vi "Excel_Insert_Control.vi"(0 "Worksheet":refnum<k7>, 1 "Excel.Shapes":refnum<k7>, 5 "Ctl Refnum":refnum<vi>, 7 "image depth":T1=3 items=["B&W", "4 bits", "8 bits", "24 bits"], 9 "image file type(.jpg)":enum16{".jpg", ".png"}(ring), 11 "error in (no error)":errorcluster, 12 "Position (Excel)":cluster{"row":i32, "column":i32}, 13 "name":string) -> (15 "error out":errorcluster)   [LabVIEW 2017, in "NI_ReportGenerationToolkit.lvlib"]
uses:
  <vilib>/addons/_office/NI_ReportGenerationToolkit.lvlib
  <vilib>/Utility/NIReport.llb/image depth.ctl
  <vilib>/Utility/NIReport.llb/NI_ReportGenerationCore.lvlib
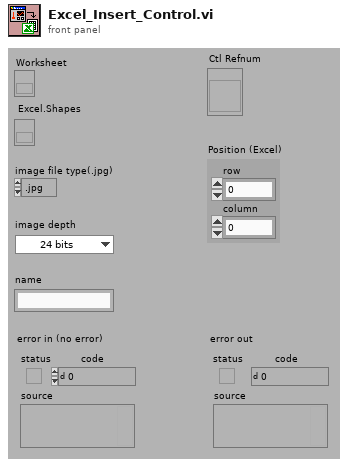
[diagram p1: front panel]
types:
  T1 = typedef "NI_ReportGenerationCore.lvlib/image depth.ctl" = u16
  T2 = typedef "imagedata.ctl" = cluster{"image type":i32, "image depth":i32, "image":u8[], "mask":u8[], "colors":u32[], "Rectangle":cluster{"left":i16, "top":i16, "right":i16, "bottom":i16}}
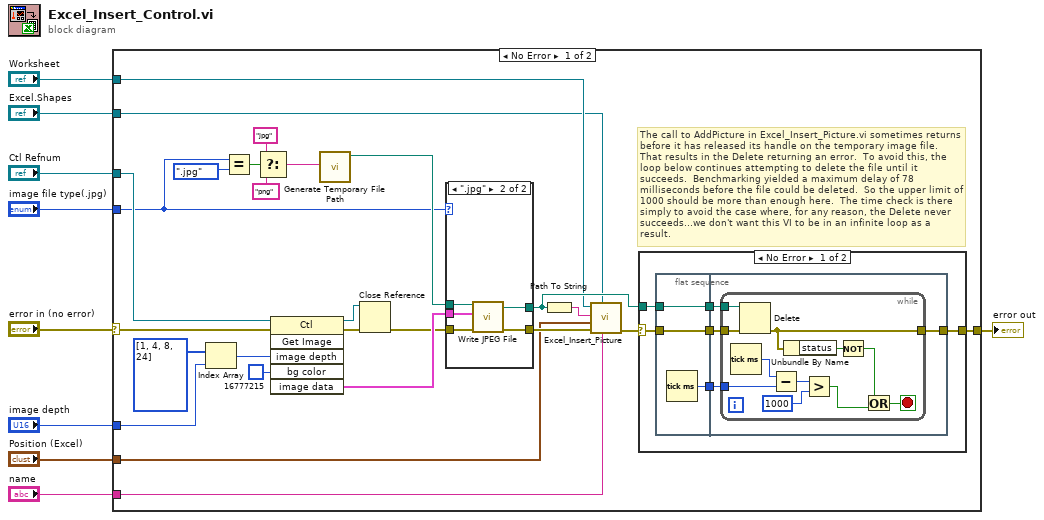
[diagram p0: block diagram]
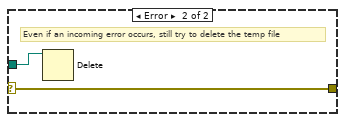
[diagram p2: hidden frame]
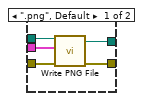
[diagram p3: hidden frame]
diagram:
  n1 = case shown="No Error" "error in (no error)" {
    selector: "error in (no error)" -> [w24 w72]
    tunnel: "image depth" -> [w34 _]
    tunnel: [w30 w72] -> w8
    tunnel: "Excel.Shapes" -> [w17 _]
    tunnel: "image file type(.jpg)" -> [w15 _]
    tunnel: "Position (Excel)" -> [w22 _]
    tunnel: "name" -> [w21 _]
    tunnel: "Worksheet" -> [w20 _]
    tunnel: "Ctl Refnum" -> [w19 _]
    frame No Error {
      # "The call to AddPicture in Excel_Insert_Picture.vi sometimes returns before it has released its handle on the temporary image file.  That results in the Delete returning an error.  To avoid this, the loop below continues attempting to delete the file until it succeeds.  Benchmarking yielded a maximum delay of 78 milliseconds before the file could be deleted.  So the upper limit of 1000 should be more than enough here.  The time check is there simply to avoid the case where, for any reason, the Delete never succeeds...we don't want this VI to be in an infinite loop as a result."
      n2 = Index Array(array=i32[] [1, 4, 8, 24] ("Array Constant"), index=w34) -> (element=w23:i32)
      n3 = Equal?(x=w15, y=enum16{".jpg", ".png"}.".jpg") -> (x = y?=w13:bool)
      n4 = Select(t="jpg", s=w13, f="png") -> (s? t:f=w12:string)
      n5 = invoke class="Ctl" method="Get Image"(reference=w19, error in=w24, "image depth"=w23, "bg color"=u32 16777215) -> (reference out=w27:refnum<vi>, error out=w26:errorcluster, "image data"=w33:T2)  [unwired: 2 in, 3 out]
      n6 = call <vilib>:"Generate Temporary File Path.vi"("Temporary File Extension (tmp)"=w12) -> ("Unique Temporary File Path"=w16:path)  [unwired: 1 in, 9 out]
      n7 = Close Reference(reference=w27, error in (no error)=w26) -> (error out=w25:errorcluster)
      n8 = case shown="\".jpg\"" w15 {
        tunnel: w33 -> [w62 w67]
        tunnel: w16 -> [w66 w71]
        tunnel: w25 -> [w65 w70]
        tunnel: [w64 w69] -> w32
        tunnel: [w63 w68] -> w29
        frame ".png", Default {
          n9 = call <vilib>:"Write PNG File.vi"("error in (no error)"=w65, "image data"=w62, "path to PNG file"=w66) -> ("error out"=w64:errorcluster, "path"=w63:path)  [unwired: 2 in, 5 out]
        }
        frame ".jpg" {
          n10 = call <vilib>:"Write JPEG File.vi"("error in (no error)"=w70, "image data"=w67, "path to JPEG file"=w71) -> ("error out"=w69:errorcluster, "path"=w68:path)  [unwired: 1 in, 6 out]
        }
      }
      n11 = Path To String(path=w29) -> (string=w31:string)
      n12 = call <vilib>:"Excel_Insert_Picture.vi"("name"=w21, "Shapes"=w17, "error in (no error)"=w32, "position"=w22, "Filename"=w31, "Worksheet"=w20) -> ("error out"=w18:errorcluster)  [unwired: 5 out]
      n13 = case shown="No Error" w18 {
        selector: w18 -> [w36 w61]
        tunnel: [w38 w61] -> w30
        tunnel: w29 -> [w37 w60]
        frame No Error {
          n14 = flat-sequence {
            tunnel: w36 -> [w43]
            tunnel: w37 -> [w44]
            tunnel: [w44] -> w41
            tunnel: [w43] -> w40
            tunnel: [w42] -> w39
            tunnel: [w48] -> w38
            tunnel: w41 -> [w47]
            tunnel: w40 -> [w46]
            tunnel: w39 -> [w45]
            frame #0 {
              n15 = Tick Count (ms)() -> (millisecond timer value=w42:u32)
            }
            frame #1 {
              n16 = while {
                tunnel: [w51] -> w48
                tunnel: w47 -> [w59]
                tunnel: w46 -> [w58]
                tunnel: w45 -> [w57]
                stop <- w53 stop-if-true
                n17 = Tick Count (ms)() -> (millisecond timer value=w56:u32)
                n18 = Delete(path (use dialog)=w59, error in=w58) -> (error out=w51:errorcluster)  [unwired: 5 out]
                n19 = Subtract(x=w56, y=w57) -> (x-y=w55:u32)
                n20 = Unbundle By Name(w51) -> ("status"=w50:bool)
                n21 = Greater?(x=w55, y=u32 1000) -> (0:w52:bool)
                n22 = Not(x=w50) -> (.not. x?=w49:bool)
                n23 = Or(x=w49, y=w52) -> (x .or. y?=w53:bool)
              }
            }
          }
        }
        frame Error {
          # "Even if an incoming error occurs, still try to delete the temp file"
          n24 = Delete(path (use dialog)=w60) -> ()  [unwired: 1 in, 6 out]
        }
      }
    }
    frame Error {
    }
  }
  "error out" <- w8
